vi "proc_markEvent.vi"(0 "event_type":i32, 1 "handle":i32) -> ()   [LabVIEW 2010]
uses:
  MWT_1.3.0_r1035/MultiWorm Tracker v1.3.0/data/MWT.dll
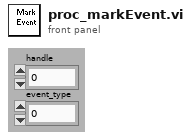
[diagram p1: front panel]
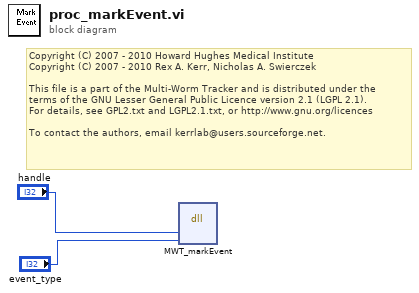
[diagram p0: block diagram]
diagram:
  # "Copyright (C) 2007 - 2010 Howard Hughes Medical Institute\nCopyright (C) 2007 - 2010 Rex A. Kerr, Nicholas A. Swierczek\n \nThis file is a part of the Multi-Worm Tracker and is distributed under the\nterms of the GNU Lesser General Public Licence version 2.1 (LGPL 2.1).\nFor details, see GPL2.txt and LGPL2.1.txt, or http://www.gnu.org/licences\n \nTo contact the authors, email kerrlab@users.sourceforge.net."
  n1 = dll-call lib="C:/Users/Marc/multi worm tracker/MWT_1.3.0_r1035/MultiWorm Tracker v1.3.0/data/MWT.dll" fn="MWT_markEvent"("handle"="handle", "event_type"="event_type") -> ()  [unwired: 6 in, 2 out]
